vi "State_Machine_Example.vi"() -> ()   [LabVIEW 2017, in "Examples.lvlib"]
uses:
  Examples.lvlib
panel:
  out "Money Deposited":string
  out "Money Deposited 3":string
  in  "Dime":bool
  out "Dispense Drink":bool
  in  "Nickel":bool
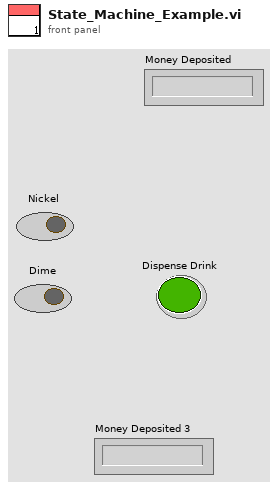
[diagram p1: front panel]
types:
  T1 = enum16{"Start", "5 cents", "10 cents", "Dispense"}
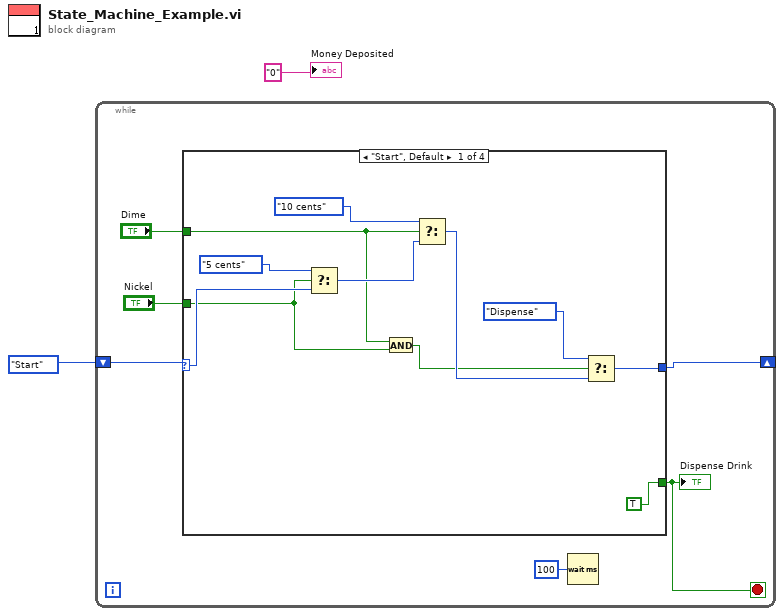
[diagram p0: block diagram]
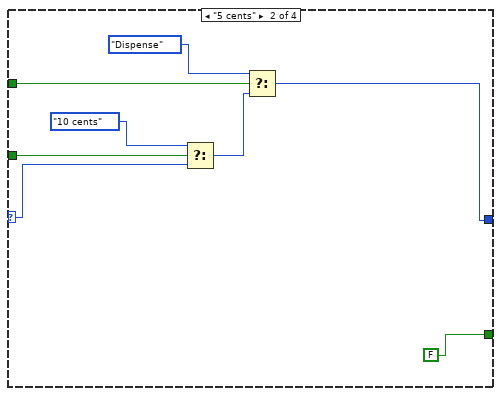
[diagram p2: hidden frame]
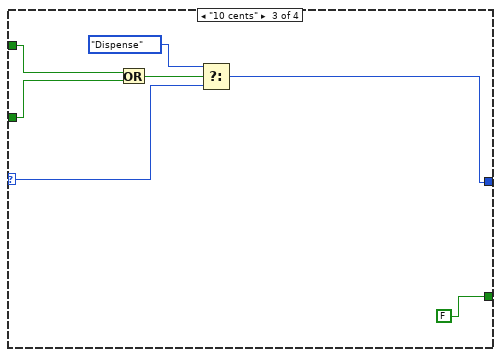
[diagram p3: hidden frame]
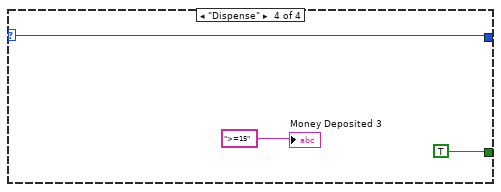
[diagram p4: hidden frame]
diagram:
  n1 = while {
    shift-right: [w5] -> _
    shift-left: T1."Start" -> [w7]
    stop <- w4 stop-if-true
    n2 = case shown="\"Start\", Default" w7 {
      selector: w7 -> [w18 w24 w30 w36]
      tunnel: "Nickel" -> [w11 w27 w33 _]
      tunnel: "Dime" -> [w12 w26 w34 _]
      tunnel: [w10 w21 w29 w36] -> w5
      tunnel: [TRUE FALSE FALSE TRUE] -> w4
      frame "Start", Default {
        n3 = Select(t=T1."5 cents", s=w11, f=w18) -> (s? t:f=w17:T1)
        n4 = And(x=w12, y=w11) -> (x .and. y?=w13:bool)
        n5 = Select(t=T1."10 cents", s=w12, f=w17) -> (s? t:f=w15:T1)
        n6 = Select(t=T1."Dispense", s=w13, f=w15) -> (s? t:f=w10:T1)
      }
      frame "5 cents" {
        n7 = Select(t=T1."10 cents", s=w27, f=w24) -> (s? t:f=w23:T1)
        n8 = Select(t=T1."Dispense", s=w26, f=w23) -> (s? t:f=w21:T1)
      }
      frame "10 cents" {
        n9 = Or(x=w34, y=w33) -> (x .or. y?=w32:bool)
        n10 = Select(t=T1."Dispense", s=w32, f=w30) -> (s? t:f=w29:T1)
      }
      frame "Dispense" {
        "Money Deposited 3" <- ">=15"
      }
    }
    "Dispense Drink" <- w4
    n11 = Wait (ms)(milliseconds to wait=u32 100) -> ()  [unwired: 1 out]
  }
  "Money Deposited" <- "0"
